vi "SP Update Formats on Measurement Changes.vi"(4 "error in (no error)":errorcluster, 5 "SNA? (F)":bool, 6 "Parameter String":string caption="Parameter", 7 "Format":refnum<vi>) -> (0 "error out":errorcluster)   [LabVIEW 2011]
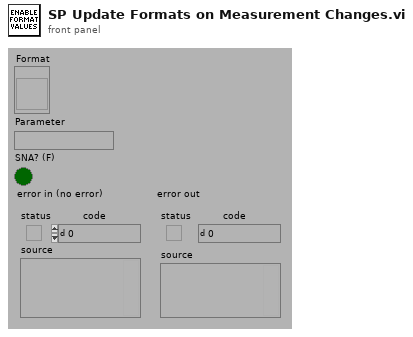
[diagram p1: front panel]
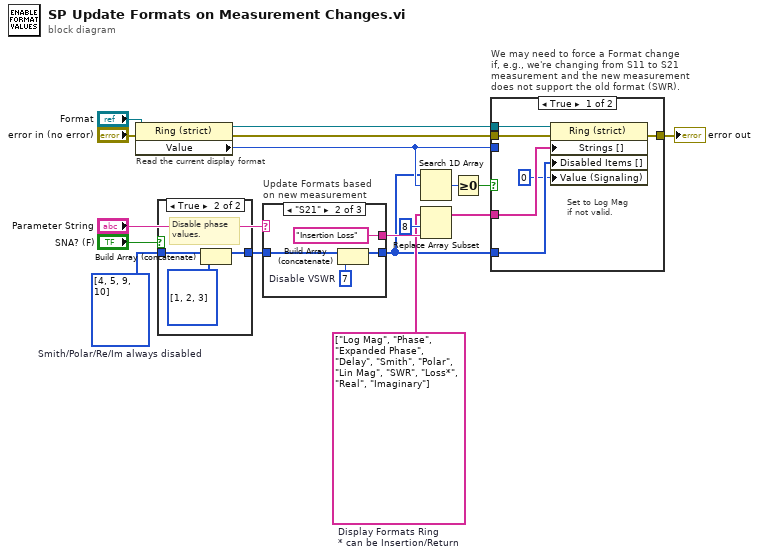
[diagram p0: block diagram]
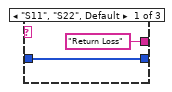
[diagram p3: hidden frame]
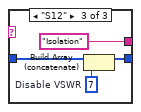
[diagram p4: hidden frame]
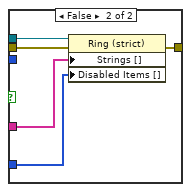
[diagram p5: hidden frame]
diagram:
  w1 = i32[] [4, 5, 9, 10]  # Smith/Polar/Re/Im always disabled
  w9 = string[] ["Log Mag", "Phase", "Expanded Phase", "Delay", "Smith", "Polar", "Lin Mag", "SWR", "Loss*", "Real", "Imaginary"]  # Display Formats Ring * can be Insertion/Return
  # "Read the current display format"
  n1 = property on="Property Node" class="Ring (strict)"(reference="Format", error in="error in (no error)") -> (reference out=w17:refnum<vi>, error out=w15:errorcluster, "Value"=w6:i32)
  n2 = case shown="True" "SNA? (F)" {
    tunnel: w1 -> [w18 w20]
    tunnel: [w18 w19] -> w2
    frame False {
    }
    frame True {
      # "Disable phase\nvalues."
      n3 = Build Array (concatenate)(w20, i32[] [1, 2, 3]) -> (w19:i32[])
    }
  }
  n4 = case "Update Formats based\non new measurement" shown="\"S21\"" "Parameter String" {
    tunnel: [w22 w26 w30] -> w3
    tunnel: ["Return Loss" "Insertion Loss" "Isolation"] -> w11
    tunnel: w2 -> [w22 w24 w28]
    frame "S11", "S22", Default {
    }
    frame "S21" {
      w27 = 7  # Disable VSWR
      n5 = Build Array (concatenate)(w24, w27) -> (w26:i32[])
    }
    frame "S12" {
      w31 = 7  # Disable VSWR
      n6 = Build Array (concatenate)(w28, w31) -> (w30:i32[])
    }
  }
  n7 = Search 1D Array(1D array=w3, element=w6) -> (index of element=w8:i32)  [unwired: 1 out]
  n8 = Replace Array Subset(array=w9, new element=w11, index=8) -> (w10:string[])
  n9 = Greater Or Equal To 0?(x=w8) -> (x >= 0?=w7:bool)
  n10 = case "We may need to force a Format change\nif, e.g., we're changing from S11 to S21\nmeasurement and the new measurement\ndoes not support the old format (SWR)." shown="True" w7 {
    tunnel: w10 -> [w37 w42]
    tunnel: w17 -> [w36 w40]
    tunnel: [w35 w39] -> w16
    tunnel: w15 -> [w34 w41]
    tunnel: w3 -> [w33 w38]
    tunnel: w6 -> [_ _]
    frame True {
      # "Set to Log Mag\nif not valid."
      n11 = property on="Property Node" class="Ring (strict)"(reference=w36, error in=w34, "Strings []"=w37, "Disabled Items []"=w33, "Value (Signaling)"=0) -> (error out=w35:errorcluster)  [unwired: 1 out]
    }
    frame False {
      n12 = property on="Property Node" class="Ring (strict)"(reference=w40, error in=w41, "Strings []"=w42, "Disabled Items []"=w38) -> (error out=w39:errorcluster)  [unwired: 1 out]
    }
  }
  "error out" <- w16
